vi "SSDCExit.vi"(4 "error in (no error)":errorcluster) -> (0 "error out":errorcluster)   [LabVIEW 2024]
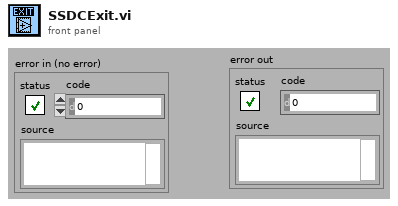
[diagram p1: front panel]
types:
  T1 = enum32{"invalid app kind", "Development System", "Run Time System", "Student Edition", "Embedded LabVIEW", "Evaluation", "Custom"}
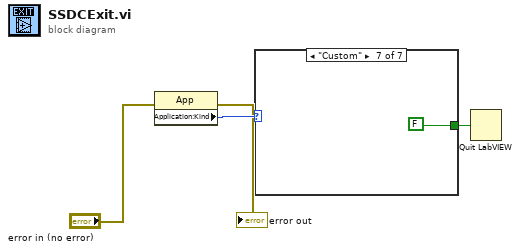
[diagram p0: block diagram]
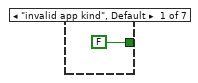
[diagram p2: hidden frame]
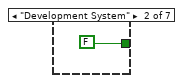
[diagram p3: hidden frame]
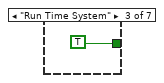
[diagram p4: hidden frame]
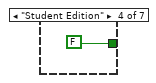
[diagram p5: hidden frame]
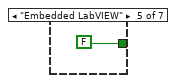
[diagram p6: hidden frame]
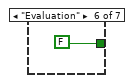
[diagram p7: hidden frame]
diagram:
  n1 = property class="App"(error in="error in (no error)") -> (error out=→"error out":errorcluster, "Application:Kind"=w4:T1)  [unwired: 1 in, 1 out]
  n2 = case shown="\"Custom\"" w4 {
    tunnel: [FALSE ("quit? (T)") FALSE ("quit? (T)") TRUE ("quit? (T)") FALSE ("quit? (T)") FALSE ("quit? (T)") FALSE ("quit? (T)") FALSE ("quit? (T)")] -> w3
    frame "invalid app kind", Default {
    }
    frame "Development System" {
    }
    frame "Run Time System" {
    }
    frame "Student Edition" {
    }
    frame "Embedded LabVIEW" {
    }
    frame "Evaluation" {
    }
    frame "Custom" {
    }
  }
  n3 = Quit LabVIEW(quit? (T)=w3) -> ()
